vi "Drop Tables.vi"() -> ()   [LabVIEW 2014, in "DB-Configuration.lvlib"]
doc: "This is a utilitiy VI to drop configuration tables in Oracle."
uses:
  DB-Configuration.lvlib
  <vilib>/addons/database/Auxilliary.llb/DB Tools Transaction.ctl
  <vilib>/addons/database/Connection.llb/DB Tools Open Connec (String).vi
  <vilib>/addons/database/Connection.llb/Conn Transaction.vi
  <vilib>/addons/database/NI_Database_API.lvlib
panel:
  out "OK?":bool
  # "Drop configuration tables in Oracle."
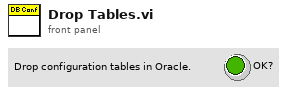
[diagram p1: front panel]
types:
  T1 = typedef "NI_Database_API.lvlib/DB Tools Transaction.ctl" = enum16{"begin", "commit", "rollback"}
  T2 = typedef "NI_Database_API.lvlib/Conn ObjectReference.ctl" = refnum<k1>
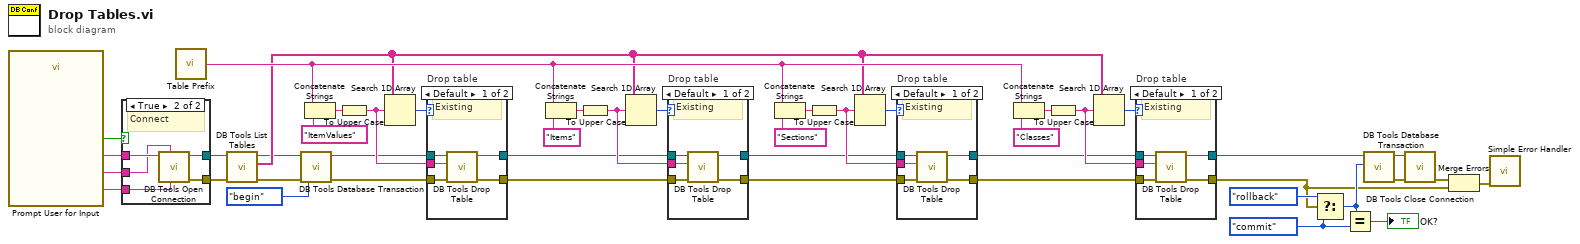
[diagram p0: block diagram]
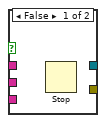
[diagram p6: hidden frame]
diagram:
  w11 = DB_Tools_Transaction."commit" ("operation (begin)")
  n1 = call "Prompt User for Input"() -> ("Password"=w42:string, "User Name"=w43:string, "ODBC Name"=w44:string, "OK"=w41:bool)  [unwired: 15 in, 1 out]
  n2 = case shown="True" w41 {
    tunnel: w44 -> [_ w49]
    tunnel: w43 -> [_ w48]
    tunnel: w42 -> [_ w47]
    tunnel: [_ w46] -> w40
    tunnel: [_ w45] -> w39
    frame False {
      n3 = Stop() -> ()  [unwired: 1 in]
    }
    frame True {
      # "Connect"
      n4 = call-poly <vilib>:"DB Tools Open Connection.vi"("password"=w47, "userID"=w48, "connection information"=w49) -> ("error out"=w45:errorcluster, "connection reference"=w46:T2)  [unwired: 5 in]
    }
  }
  n5 = call "Table Prefix.vi"() -> ("DB Table Prefix"=w19:string)
  n6 = call <vilib>:"DB Tools List Tables.vi"("error in (no error)"=w39, "connection reference"=w40) -> ("error out"=w3:errorcluster, "tables"=w18:string[], "connection reference out"=w5:T2)  [unwired: 3 in]
  n7 = call-poly <vilib>:"DB Tools Database Transaction.vi"("error in (no error)"=w3, "operation (begin)"=DB_Tools_Transaction."begin", "connection reference"=w5) -> ("error out"=w2:errorcluster, "connection reference out"=w4:T2)  [unwired: 3 in]
  n8 = Concatenate Strings(w19, "ItemValues" ("table")) -> (w36:string)
  n9 = To Upper Case(1:w36) -> (0:w35:string)
  n10 = Search 1D Array(1D array=w18, element=w35) -> (index of element=w38:i32)  [unwired: 1 in]
  n11 = case "Drop table" shown="Default" w38 {
    tunnel: w4 -> [w54 w56]
    tunnel: w2 -> [w53 w55]
    tunnel: w35 -> [w52 _]
    tunnel: [w51 w56] -> w31
    tunnel: [w50 w55] -> w30
    frame Default {
      # "Existing"
      n12 = call <vilib>:"DB Tools Drop Table.vi"("error in (no error)"=w53, "table"=w52, "connection reference"=w54) -> ("error out"=w50:errorcluster, "connection reference out"=w51:T2)  [unwired: 5 in]
    }
    frame -1 {
      # "Not existing"
    }
  }
  n13 = Concatenate Strings(w19, "Items" ("table")) -> (w33:string)
  n14 = To Upper Case(1:w33) -> (0:w34:string)
  n15 = Search 1D Array(1D array=w18, element=w34) -> (index of element=w32:i32)  [unwired: 1 in]
  n16 = case "Drop table" shown="Default" w32 {
    tunnel: w31 -> [w61 w63]
    tunnel: w30 -> [w60 w62]
    tunnel: w34 -> [w59 _]
    tunnel: [w58 w63] -> w26
    tunnel: [w57 w62] -> w25
    frame Default {
      # "Existing"
      n17 = call <vilib>:"DB Tools Drop Table.vi"("error in (no error)"=w60, "table"=w59, "connection reference"=w61) -> ("error out"=w57:errorcluster, "connection reference out"=w58:T2)  [unwired: 5 in]
    }
    frame -1 {
      # "Not existing"
    }
  }
  n18 = Concatenate Strings(w19, "Sections" ("table")) -> (w28:string)
  n19 = To Upper Case(1:w28) -> (0:w27:string)
  n20 = Search 1D Array(1D array=w18, element=w27) -> (index of element=w29:i32)  [unwired: 1 in]
  n21 = case "Drop table" shown="Default" w29 {
    tunnel: w26 -> [w68 w70]
    tunnel: w25 -> [w67 w69]
    tunnel: w27 -> [w66 _]
    tunnel: [w65 w70] -> w21
    tunnel: [w64 w69] -> w20
    frame Default {
      # "Existing"
      n22 = call <vilib>:"DB Tools Drop Table.vi"("error in (no error)"=w67, "table"=w66, "connection reference"=w68) -> ("error out"=w64:errorcluster, "connection reference out"=w65:T2)  [unwired: 5 in]
    }
    frame -1 {
      # "Not existing"
    }
  }
  n23 = Concatenate Strings(w19, "Classes" ("table")) -> (w23:string)
  n24 = To Upper Case(1:w23) -> (0:w24:string)
  n25 = Search 1D Array(1D array=w18, element=w24) -> (index of element=w22:i32)  [unwired: 1 in]
  n26 = case "Drop table" shown="Default" w22 {
    tunnel: w21 -> [w75 w77]
    tunnel: w20 -> [w74 w76]
    tunnel: w24 -> [w73 _]
    tunnel: [w72 w77] -> w8
    tunnel: [w71 w76] -> w6
    frame Default {
      # "Existing"
      n27 = call <vilib>:"DB Tools Drop Table.vi"("error in (no error)"=w74, "table"=w73, "connection reference"=w75) -> ("error out"=w71:errorcluster, "connection reference out"=w72:T2)  [unwired: 5 in]
    }
    frame -1 {
      # "Not existing"
    }
  }
  n28 = Select(t=DB_Tools_Transaction."rollback" ("operation (begin)"), s=w6, f=w11) -> (s? t:f=w12:T1)
  n29 = Equal?(x=w12, y=w11) -> (x = y?=→"OK?":bool)
  n30 = call-poly <vilib>:"DB Tools Database Transaction.vi"("operation (begin)"=w12, "connection reference"=w8) -> ("error out"=w9:errorcluster)  [unwired: 4 in, 1 out]
  n31 = call <vilib>:"DB Tools Close Connection.vi"("error in (no error)"=w9, "connection reference"=w8) -> ("error out"=w37:errorcluster)  [unwired: 5 in]
  n32 = Merge Errors(w37, w6) -> (w7:errorcluster)
  n33 = call <vilib>:"Simple Error Handler.vi"("error in (no error)"=w7) -> ()  [unwired: 4 in, 5 out]
